vi "ClearAllErrorLog.vi"() -> ()   [LabVIEW 2019]
panel:
  out "error out":errorcluster
  in  "Error In":errorcluster
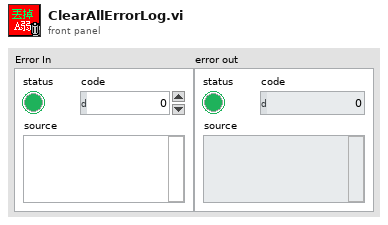
[diagram p1: front panel]
types:
  T1 = enum16{"open", "replace", "create", "open or create", "replace or create", "replace or create with confirmation"}
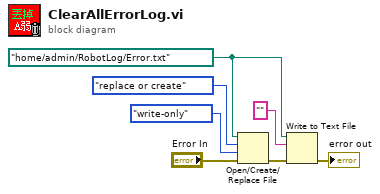
[diagram p0: block diagram]
diagram:
  w2 = path "/home/admin/RobotLog/Error.txt" ("file path (dialog if empty)")
  n1 = Open/Create/Replace File(file path (use dialog)=w2, error in="Error In", operation (0:open)=T1."replace or create", access (0:read/write)=enum16{"read/write", "read-only", "write-only"}."write-only") -> (error out=w4:errorcluster)  [unwired: 2 in, 2 out]
  n2 = Write to Text File(file (use dialog)=w2, text="", error in=w4) -> (error out=→"error out":errorcluster)  [unwired: 1 in, 2 out]
